vi "DiscArchiver.ProcEvents.vi"(0 "i ref in":refnum<vi>, 5 "error in (no error)":errorcluster) -> (14 "i ref out":refnum<vi>, 19 "error out":errorcluster)   [LabVIEW 2014, in "DiscArchiver.lvlib"]
doc: "This method is used to define the events the object will listen to. Add your own events here."
uses:
  DiscArchiver.lvlib
  CSCore/BaseProcess/BaseProcess.event definition.ctl
  CSCore/CAEObj/CAEObj.event definition.ctl
  CSCore/BaseProcess/BaseProcess.descriptor string definition.ctl
  CSCore/BaseProcess/BaseProcess.lvlib
  CSCore/CAEObj/CAEObj.lvlib
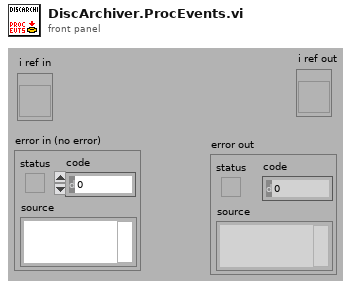
[diagram p1: front panel]
types:
  T1 = typedef "BaseProcess.lvlib/BaseProcess.event definition.ctl" = cluster{"CAEEvtDef":T2, "Data Descriptor":T3}
  T2 = typedef "CAEObj.lvlib/CAEObj.event definition.ctl" = cluster{"URL":string, "enable":bool, "ignoreResID":bool}
  T3 = typedef "BaseProcess.lvlib/BaseProcess.descriptor string definition.ctl" = string
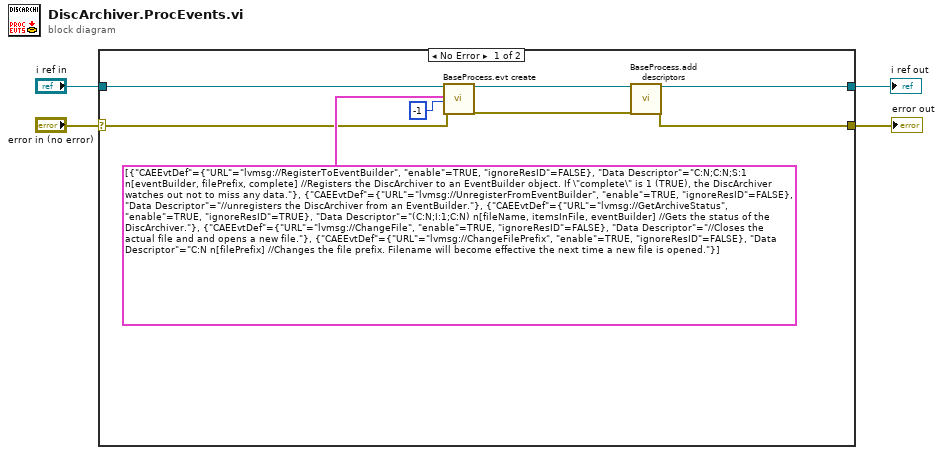
[diagram p0: block diagram]
diagram:
  n1 = case shown="No Error" "error in (no error)" {
    selector: "error in (no error)" -> [w5 w13]
    tunnel: "i ref in" -> [w12 w14]
    tunnel: [w10 w14] -> w3
    tunnel: [w8 w13] -> w2
    frame No Error {
      n2 = call "BaseProcess.evt create.vi"("i ref in"=w12, "newEvents"=T1[] [{"CAEEvtDef"={"URL"="lvmsg://RegisterToEventBuilder", "enable"=TRUE, "ignoreResID"=FALSE}, "Data Descriptor"="C:N;C:N;S:1 n[eventBuilder, filePrefix, complete] //Registers the DiscArchiver to an EventBuilder object. If \"complete\" is 1 (TRUE), the DiscArchiver watches out not to miss any data."}, {"CAEEvtDef"={"URL"="lvmsg://UnregisterFromEventBuilder", "enable"=TRUE, "ignoreResID"=FALSE}, "Data Descriptor"="//unregisters the DiscArchiver from an EventBuilder."}, {"CAEEvtDef"={"URL"="lvmsg://GetArchiveStatus", "enable"=TRUE, "ignoreResID"=TRUE}, "Data Descriptor"="(C:N;I:1;C:N) n[fileName, itemsInFile, eventBuilder] //Gets the status of the DiscArchiver."}, {"CAEEvtDef"={"URL"="lvmsg://ChangeFile", "enable"=TRUE, "ignoreResID"=FALSE}, "Data Descriptor"="//Closes the actual file and and opens a new file."}, {"CAEEvtDef"={"URL"="lvmsg://ChangeFilePrefix", "enable"=TRUE, "ignoreResID"=FALSE}, "Data Descriptor"="C:N n[filePrefix] //Changes the file prefix. Filename will become effective the next time a new file is opened."}] ("new events"), "ms timeout (10000)"=-1, "error in (no error)"=w5) -> ("i ref out"=w11:refnum<vi>, "error out"=w9:errorcluster)  [unwired: 12 in, 2 out]
      n3 = call "BaseProcess.add descriptors.vi"("i ref in"=w11, "error in (no error)"=w9) -> ("i ref out"=w10:refnum<vi>, "error out"=w8:errorcluster)  [unwired: 15 in, 1 out]
    }
    frame Error {
    }
  }
  "i ref out" <- w3
  "error out" <- w2
